vi "Rotations to encoder.vi"(10 "Rotations":dbl) -> (2 "Encoder counts":dbl)   [LabVIEW 2017]
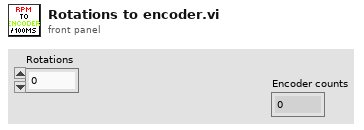
[diagram p1: front panel]
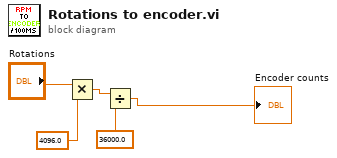
[diagram p0: block diagram]
diagram:
  n1 = Multiply(x="Rotations", y=4096.0) -> (x*y=w3:dbl)
  n2 = Divide(x=w3, y=36000.0) -> (x/y=→"Encoder counts":dbl)
